vi "Read A&E Type.vi"(8 "error in (no error)":errorcluster, 11 "AE in":refnum<class "AE.lvclass">) -> (0 "error out":errorcluster, 2 "A&E Type":T1, 3 "AE out":refnum<class "AE.lvclass">)   [LabVIEW 2015, in "CS++ProcessVariables.lvlib" / "AE.lvclass"]
doc: "Read attribute value."
uses:
  AE.lvclass
  AE Type.ctl
  AE.lvclass/AE.ctl
  CS++ProcessVariables.lvlib
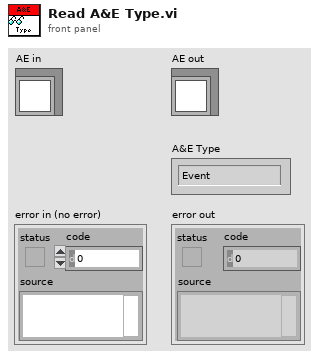
[diagram p1: front panel]
types:
  T1 = typedef "CS++ProcessVariables.lvlib/AE Type.ctl" = enum16{"Event", "HI_HI", "HI", "LO", "LO_LO", "Boolean", "ROC", "Invalid", "Other"}
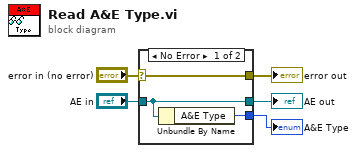
[diagram p0: block diagram]
diagram:
  n1 = case shown="No Error" "error in (no error)" {
    selector: "error in (no error)" -> [w8 w9]
    tunnel: [w8 w9] -> w4
    tunnel: [w7 w10] -> w2
    tunnel: "AE in" -> [w7 w10]
    tunnel: [w6 _] -> w1
    frame No Error {
      n2 = Unbundle By Name(w7) -> ("A&E Type"=w6:T1)
    }
    frame Error {
    }
  }
  "error out" <- w4
  "AE out" <- w2
  "A&E Type" <- w1
